vi "Test To Report Entry.vi"(8 "error in (no error)":errorcluster, 10 "Test Node":T1, 11 "Basic Test Manager in":refnum<class "Basic Test Manager.lvclass">) -> (0 "error out":errorcluster, 2 "String":string, 3 "Basic Test Manager out":refnum<class "Basic Test Manager.lvclass">)   [LabVIEW 2009, in "Caraya.lvlib" / "Basic Test Manager.lvclass"]
uses:
  Basic Test Manager.lvclass
  Test Event Storage/Test Node.ctl
  Test Registration Data.ctl
  Test Event Storage/Test Event Storage.lvclass
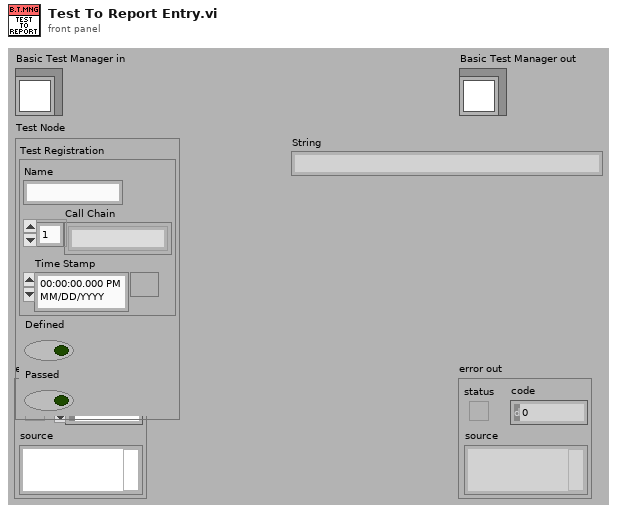
[diagram p1: front panel]
types:
  T1 = typedef "Caraya.lvlib/Test Event Storage.lvclass/Test Node.ctl" = cluster{"Test Registration":T2, "Defined":bool, "Passed":bool}
  T2 = typedef "Caraya.lvlib/Basic Test Manager.lvclass/Test Registration Data.ctl" = cluster{"Name":string, "Call Chain":string[], "Time Stamp":timestamp}
  T3 = typedef "Caraya.lvlib/Basic Test Manager.lvclass/Test State.ctl" = enum16{"Empty", "Unknown", "Fail", "Pass", "Skip", "Error"}
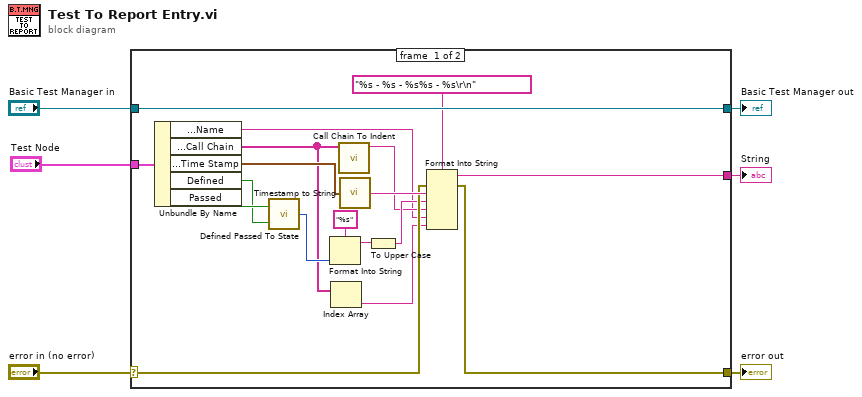
[diagram p0: block diagram]
diagram:
  n1 = case shown="No Error" "error in (no error)" {
    selector: "error in (no error)" -> [w17 w26]
    tunnel: [w16 w26] -> w5
    tunnel: [w24 w25] -> w3
    tunnel: "Basic Test Manager in" -> [w24 w25]
    tunnel: "Test Node" -> [w23 _]
    tunnel: [w7 _] -> w1
    frame #0 {
      n2 = Unbundle By Name(w23) -> ("Test Registration.Name"=w9:string, "Test Registration.Call Chain"=w10:string[], "Test Registration.Time Stamp"=w20:timestamp, "Defined"=w21:bool, "Passed"=w22:bool)
      n3 = call "Defined Passed To State.vi"("Defined"=w21, "Passed"=w22) -> ("State"=w15:T3)
      n4 = Format Into String(format string="%s", w15) -> (resulting string=w13:string)  [unwired: 2 in, 1 out]
      n5 = Index Array(array=w10) -> (element=w8:string)  [unwired: 1 in]
      n6 = call "Call Chain To Indent.vi"("Call Chain"=w10) -> ("Indent"=w11:string)  [unwired: 10 in]
      n7 = call "Timestamp to String.vi"("Time Stamp"=w20) -> ("date/time string"=w19:string)
      n8 = To Upper Case(1:w13) -> (0:w12:string)
      n9 = Format Into String(format string="%s - %s - %s%s - %s\r\n", error in=w17, w19, w12, w11, w9, w8) -> (resulting string=w7:string, error out=w16:errorcluster)  [unwired: 1 in]
    }
    frame #1 {
    }
  }
  "error out" <- w5
  "Basic Test Manager out" <- w3
  "String" <- w1
